vi "Negan.vi"() -> ()   [LabVIEW 2016]
panel:
  out "String":string
  in  "frases":T1(ring)
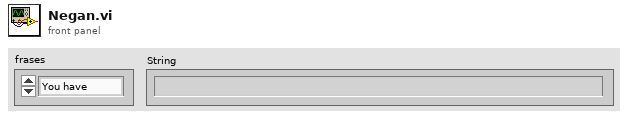
[diagram p1: front panel]
types:
  T1 = enum16{"You have", "Lucille", "You can breath", "Little", "I simply"}
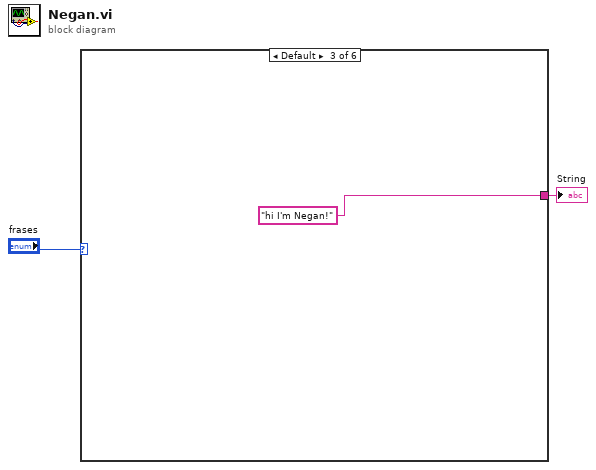
[diagram p0: block diagram]
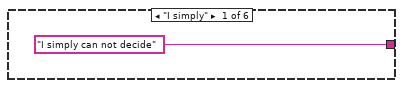
[diagram p2: hidden frame]
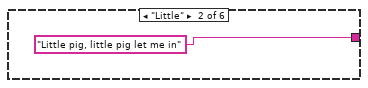
[diagram p3: hidden frame]
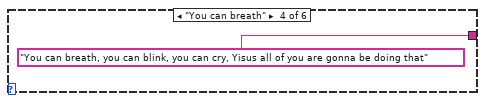
[diagram p4: hidden frame]
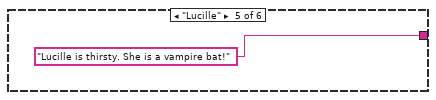
[diagram p5: hidden frame]
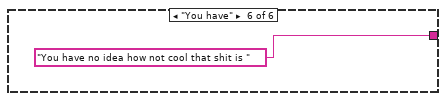
[diagram p6: hidden frame]
diagram:
  n1 = case shown="Default" "frases" {
    tunnel: ["I simply can not decide" "Little pig, little pig let me in" "hi I'm Negan!" "You can breath, you can blink, you can cry, Yisus all of you are gonna be doing that" "Lucille is thirsty. She is a vampire bat!" "You have no idea how not cool that shit is "] -> w1
    frame "I simply" {
    }
    frame "Little" {
    }
    frame Default {
    }
    frame "You can breath" {
    }
    frame "Lucille" {
    }
    frame "You have" {
    }
  }
  "String" <- w1
